vi "RaspCode.vi"   [LabVIEW 2020]
uses:
  <vilib>/MakerHub/LINX/Public/Peripherals/Digital/Digital Write N Chans.vi
  <vilib>/MakerHub/LINX/Private/Local IO/LinxDigitalWrite.vi
  <vilib>/MakerHub/LINX/Public/Utilities/Check Channel.vi
  <vilib>/MakerHub/LINX/Private/Local IO/Handle Errors.vi
  <vilib>/MakerHub/LINX/Public/Utilities/Open Local.vi
  <vilib>/MakerHub/LINX/Private/Utilties/Generate Error.vi
  <vilib>/MakerHub/LINX/LMH-LINX.lvlib
types:
  T1 = typedef "LMH-LINX.lvlib/LINX Ref.ctl" = cluster{"IO":T2, "Interface":T3, "LINX Device Config":T4}
  T2 = typedef "LMH-LINX.lvlib/Platform.ctl" = enum16{"Remote", "Local"}
  T3 = typedef "LMH-LINX.lvlib/Interface.ctl" = enum16{"Serial", "TCP"}
  T4 = typedef "LMH-LINX.lvlib/Device.lvlib/LINX Device Config.ctl" = cluster{"Interface":T3, "COM Port":refnum<visa-resource-name>, "TCP Configuration":T5, "Device Family":u8, "Device ID":u8, "Device Name":string, "TCP Ref":refnum<k5>, "Channels":T6}
  T5 = typedef "LMH-LINX.lvlib/Device.lvlib/TCP Config.ctl" = cluster{"IP Address":string, "Port":u16}
  T6 = typedef "LMH-LINX.lvlib/Channels.ctl" = cluster{"DI":u8[], "DO":u8[], "AI":u8[], "AO":u8[], "PWM":u8[], "QE":u8[], "UART":u8[], "I2C 2":u8[], "SPI":u8[], "CAN":u8[], "Servo":u8[], "AI Ref (V)":dbl, "AI Resolution (Bits)":u8, "AO Ref (V)":dbl, "AO Resolution (Bits)":u8}
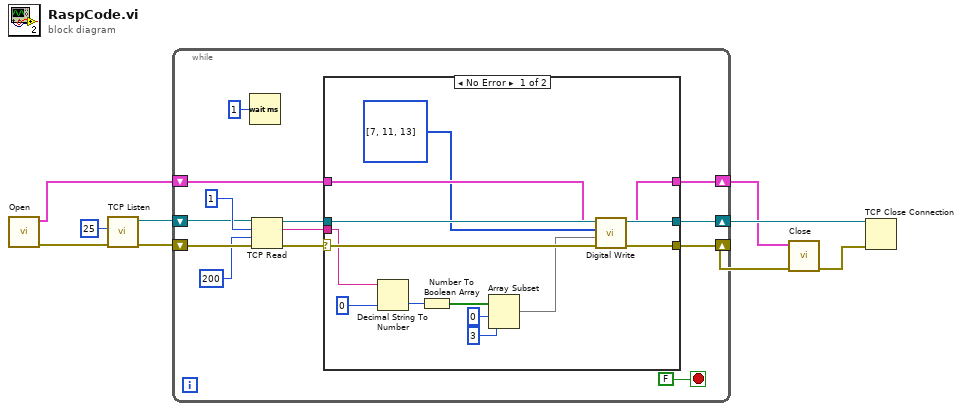
[diagram p0: block diagram]
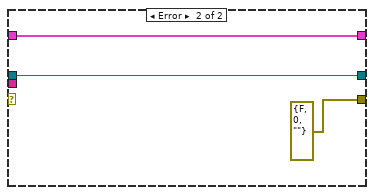
[diagram p2: hidden frame]
diagram:
  n1 = call-poly <vilib>:"Open.vi"() -> ("Error Out"=w5:errorcluster, "LINX Resource"=w4:T1)  [unwired: 9 in, 1 out]
  n2 = call <vilib>:"TCP Listen.vi"("error in (no error)"=w5, "port"=u16 25) -> ("error out"=w9:errorcluster, "connection ID"=w8:refnum<k5>)  [unwired: 5 in, 3 out]
  n3 = while {
    shift-right: [w17] -> w6
    shift-left: w8 -> [w18]
    shift-right: [w16] -> w2
    shift-left: w9 -> [w22]
    shift-right: [w13] -> w3
    shift-left: w4 -> [w14]
    stop <- FALSE stop-if-true
    n4 = Wait (ms)(milliseconds to wait=u32 1) -> ()  [unwired: 1 out]
    n5 = TCP Read(connection ID=w18, bytes to read=1, error in (no error)=w22, 9:200 ("timeout ms (25000)")) -> (connection ID out=w19:refnum<k5>, data out=w11:string, error out=w12:errorcluster)  [unwired: 1 in]
    n6 = case shown="No Error" w12 {
      selector: w12 -> [w32 _]
      tunnel: w19 -> [w35 w38]
      tunnel: [w31 errorcluster {"status"=FALSE, "code"=0, "source"=""} ("error IO")] -> w16
      tunnel: [w35 w38] -> w17
      tunnel: w14 -> [w34 w36]
      tunnel: [w33 w36] -> w13
      tunnel: w11 -> [w23 _]
      frame No Error {
        n7 = Decimal String To Number(string=w23, default (0L)=u32 0 ("default (0 I32)")) -> (number=w29:u32)  [unwired: 1 in, 1 out]
        n8 = Number To Boolean Array(number=w29) -> (Boolean array=w27:bool[])
        n9 = Array Subset "Array Subset"(array=w27, index=0, length=3) -> (w24:bool[])
        n10 = call-poly <vilib>:"Digital Write.vi"("Error In"=w32, "Values"=w24, "DO Channels"=u8[] [7, 11, 13], "LINX Resource"=w34) -> ("Error Out"=w31:errorcluster, "LINX Resource"=w33:T1)  [unwired: 6 in]
      }
      frame Error {
      }
    }
  }
  n11 = call <vilib>:"Close.vi"("Error In"=w2, "LINX Resource"=w3) -> ("Error Out"=w1:errorcluster)  [unwired: 9 in]
  n12 = TCP Close Connection(connection ID=w6, error in (no error)=w1) -> ()  [unwired: 1 in, 2 out]
